vi "ErrorCodesAndDescriptions.vi"() -> (1 "Error Descriptions":string[](array[string]), 2 "Error Names":string[](array[string])=["Event Manager error", "Invalid user event", "Invalid user event"], 3 "Error Codes":i32[](array[numeric]))   [LabVIEW 2009, in "EventManagerLibrary.lvlib" / "EventManagerErrors.lvclass"]
doc: "Defines the error codes, titles, and descriptions used by the event manager library."
uses:
  EventManagerErrors.lvclass
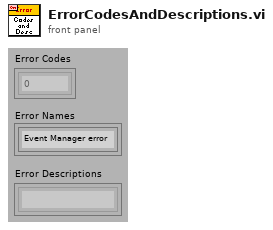
[diagram p1: front panel]
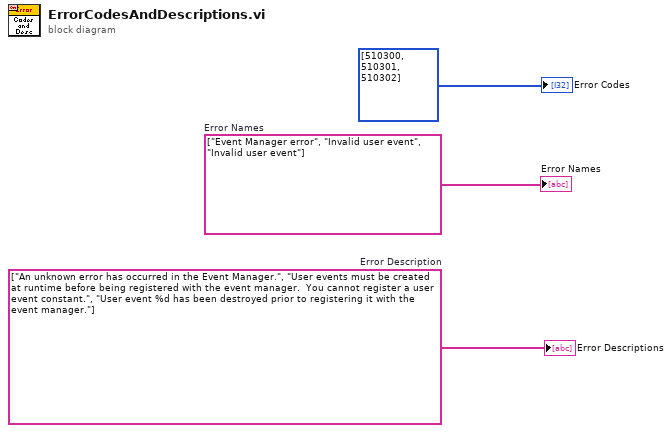
[diagram p0: block diagram]
diagram:
  w2 = string[] ["An unknown error has occurred in the Event Manager.", "User events must be created at runtime before being registered with the event manager.  You cannot register a user event constant.", "User event %d has been destroyed prior to registering it with the event manager."]  # Error Description
  w1 = string[] ["Event Manager error", "Invalid user event", "Invalid user event"]  # Error Names
  "Error Codes" <- i32[] [510300, 510301, 510302] ("Error Codes")
  "Error Descriptions" <- w2
  "Error Names" <- w1
